vi "Add State Frame.vi"(8 "error in (no error)":errorcluster, 9 "index(-1, use same group)":i32=-1, 10 "element":string, 11 "CSM-Helper in":refnum<class "CSM-Helper.lvclass">) -> (0 "error out":errorcluster, 1 "Add Frame":refnum<vi>, 3 "CSM-Helper out":refnum<class "CSM-Helper.lvclass">)   [LabVIEW 2017, in "CSM-Helper.lvclass"]
doc: "### Add State Frame.vi\n\n-- <b>Controls</b> --\n- <b>index(-1, use same group)</b>:\n- <b>element</b>:\n- <b>CSM-Helper in</b>: CSMHelper input\n\n-- <b>Indicators</b> --\n- <b>Add Frame</b>:\n- <b>CSM-Helper out</b>: CSMHelper output"
uses:
  CSM-Helper.lvclass
  CSM-Helper.lvclass/CSM-Helper.ctl
  Properties/Read Case Structure Ref.vi
  Utility/_Support/CaseStructure.llb/csmHelper-CaseStructure.lvlib
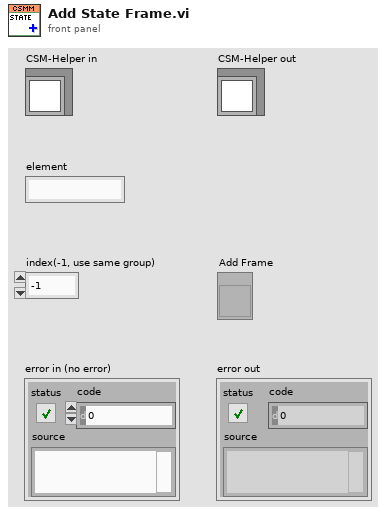
[diagram p1: front panel]
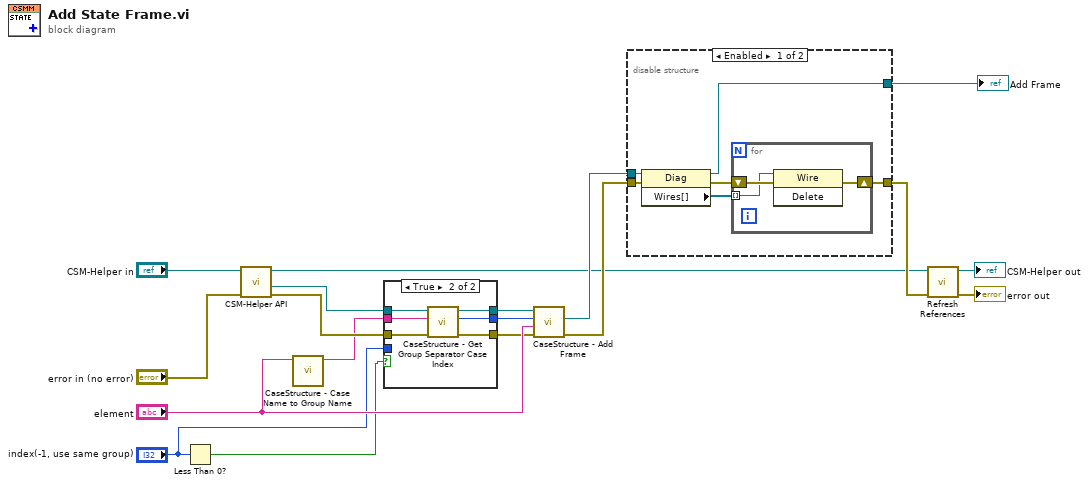
[diagram p0: block diagram]
diagram:
  n1 = Less Than 0?(x="index(-1, use same group)") -> (x < 0?=w2:bool)
  n2 = call-poly "CSM-Helper API.vi"("error in (no error)"="error in (no error)", "CSM-Helper in"="CSM-Helper in") -> ("error out"=w13:errorcluster, "Case Structure"=w3:refnum<vi>, "CSM-Helper out"=w11:refnum<class "CSM-Helper.lvclass">)  [unwired: 7 in]
  n3 = call "CaseStructure - Case Name to Group Name.vi"("element"="element") -> ("String"=w8:string)  [unwired: 10 in]
  n4 = case shown="True" w2 {
    tunnel: w13 -> [w19 w27]
    tunnel: w8 -> [_ w26]
    tunnel: [w21 w25] -> w7
    tunnel: [w20 w24] -> w6
    tunnel: [w19 w23] -> w5
    tunnel: w3 -> [w20 w22]
    tunnel: "index(-1, use same group)" -> [w21 _]
    frame False {
    }
    frame True {
      n5 = call "CaseStructure - Get Group Separator Case Index.vi"("error in (no error)"=w27, "Group Name"=w26, "CaseStructure in"=w22) -> ("error out"=w23:errorcluster, "Numeric"=w25:i32, "CaseStructure out"=w24:refnum<vi>)  [unwired: 6 in]
    }
  }
  n6 = call "CaseStructure - Add Frame.vi"("error in (no error)"=w5, "Case Name"="element", "Reference Frame Index"=w7, "CaseStructure in"=w6) -> ("error out"=w14:errorcluster, "Add Frame"=w16:refnum<vi>)  [unwired: 5 in, 1 out]
  n7 = disable-structure shown="Enabled" {
    disable-tunnel: [w33 w37] -> w17
    disable-tunnel: w16 -> [w32 w37]
    disable-tunnel: [w31 w38] -> w15
    disable-tunnel: w14 -> [w30 w38]
    frame Enabled {
      n8 = property on="Property Node" class="Diag"(reference=w32, error in=w30) -> (reference out=w33:refnum<vi>, error out=w28:errorcluster, "Wires[]"=w29:refnum<vi>[])
      n9 = for {
        shift-right: [w36] -> w31
        shift-left: w28 -> [w35]
        tunnel: w29 -> [w34] mode=indexing
        n10 = invoke class="Wire" method="Delete"(reference=w34, error in=w35) -> (error out=w36:errorcluster)  [unwired: 1 in, 2 out]
      }
    }
    frame Disabled {
    }
  }
  "Add Frame" <- w17
  n11 = call "Refresh References.vi"("error in (no error)"=w15, "CSM-Helper in"=w11) -> ("error out"=→"error out":errorcluster, "CSM-Helper out"=→"CSM-Helper out":refnum<class "CSM-Helper.lvclass">)  [unwired: 8 in]
